vi "Untitled 1.vi"() -> ()   [LabVIEW 2018]
uses:
  <vilib>/Utility/file.llb/Read Delimited Spreadsheet (DBL).vi
  PublicSubVI/Class/Sig2MS/Sig2MS.lvclass
panel:
  in  "max":dbl
  in  "min":dbl
  in  "error in (no error)":errorcluster
  in  "File Path":path
  in  "tabCtrl":T1(tab)
  in  "scriptUpd":bool
  in  "Script":string
  out "rawGraph":cluster{"x":dbl[], "y":dbl[]}(graph)
  out "diffGraph":cluster{"x":dbl[], "y":dbl[]}(graph)
  out "diffSgolayGraph":cluster{"x":dbl[], "y":dbl[]}(graph)
  out "diffConvolveGraph":cluster{"x":dbl[], "y":dbl[]}(graph)
  out "richardsonGraph":cluster{"x":dbl[], "y":dbl[]}(graph)
  out "richardsonSgolayGraph":cluster{"x":dbl[], "y":dbl[]}(graph)
  out "richardsonConvolveGraph":cluster{"x":dbl[], "y":dbl[]}(graph)
  out "sgolayGraph":cluster{"x":dbl[], "y":dbl[]}(graph)
  out "sgolaySgolayGraph":cluster{"x":dbl[], "y":dbl[]}(graph)
  out "sgolayConvolveGraph":cluster{"x":dbl[], "y":dbl[]}(graph)
  out "sgolayAdvGraph":cluster{"x":dbl[], "y":dbl[]}(graph)
  out "sgolayAdvSgolayGraph":cluster{"x":dbl[], "y":dbl[]}(graph)
  out "sgolayAdvConvolveGraph":cluster{"x":dbl[], "y":dbl[]}(graph)
  out "xyGraph":cluster{"x":dbl[], "y":dbl[]}[](graph)
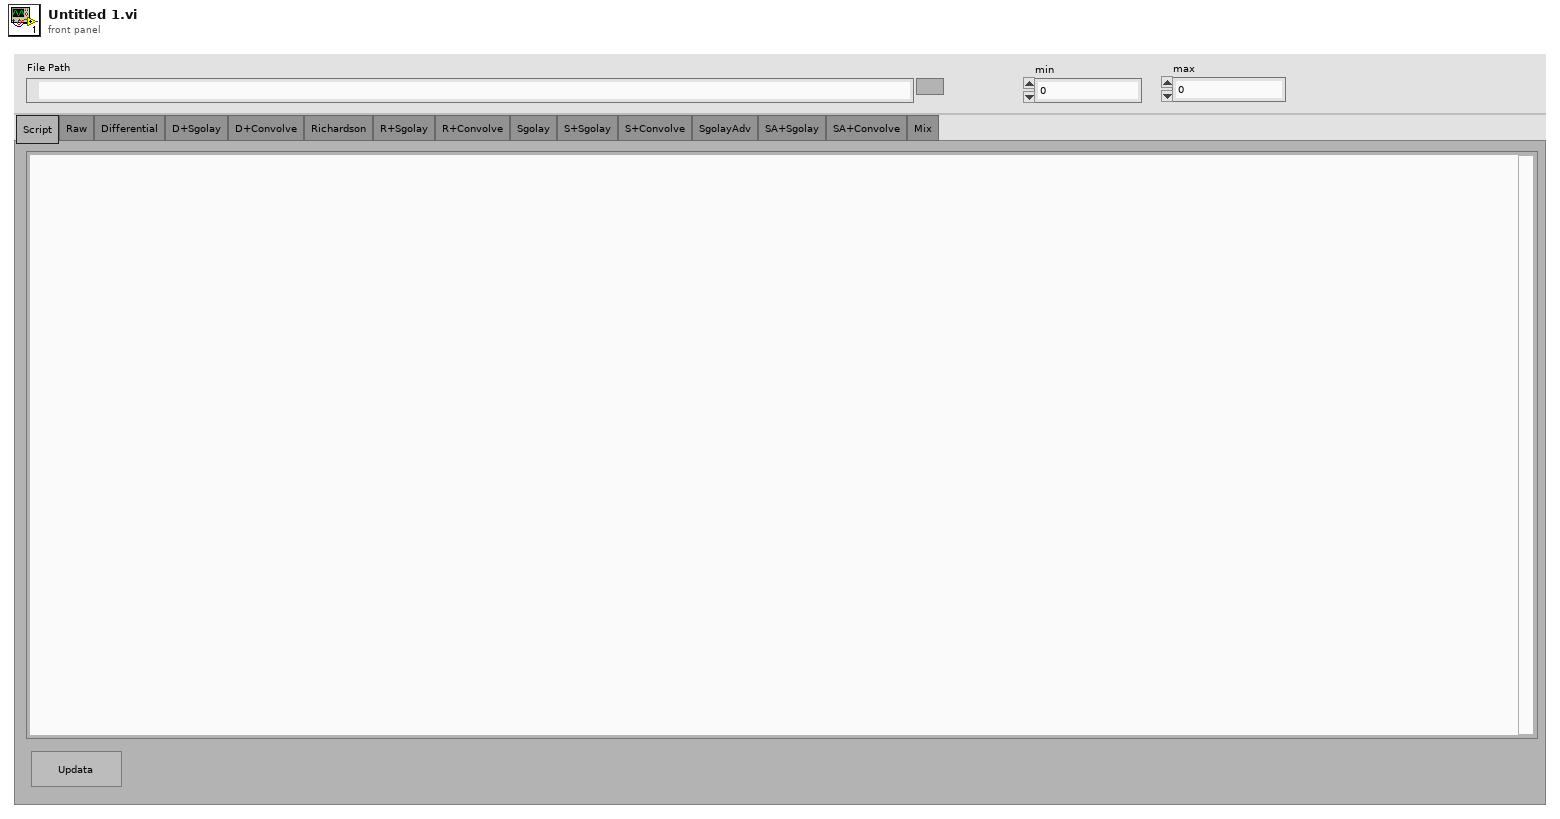
[diagram p1: front panel]
types:
  T1 = enum32{"Script", "Raw", "Differential", "D+Sgolay", "D+Convolve", "Richardson", "R+Sgolay", "R+Convolve", "Sgolay", "S+Sgolay", "S+Convolve", "SgolayAdv", "SA+Sgolay", "SA+Convolve", "Mix"}
  T2 = cluster{"startTime":dbl, "scanSig":cluster{"priDt":dbl, "priXData":dbl[], "priYData":sgl[], "beta":dbl[]}[], "ionSig":cluster{"secDt":dbl, "secYData":sgl[]}[]}
  T3 = enum16{"init", "loadScript", "newScript", "runScript", "close"}
  T4 = cluster{"priDt":dbl, "priXData":dbl[], "priYData":sgl[], "beta":dbl[]}[]
  T5 = cluster{"priDt":dbl, "priXData":dbl[], "priYData":sgl[], "beta":dbl[]}
  T6 = cluster{"startTime":dbl, "scanData":cluster{"dt":dbl, "xdata":dbl[], "ydata":sgl[], "beta":dbl[]}[], "xyXLabel":string, "xyYLabel":string, "wfmXLabel":string, "wfmYLabel":string, "ionData":cluster{"dt":dbl, "ydata":sgl[]}[], "ionXLabel":string, "ionYLabel":string}
  T7 = cluster{"dt":dbl, "xdata":dbl[], "ydata":sgl[], "beta":dbl[]}[]
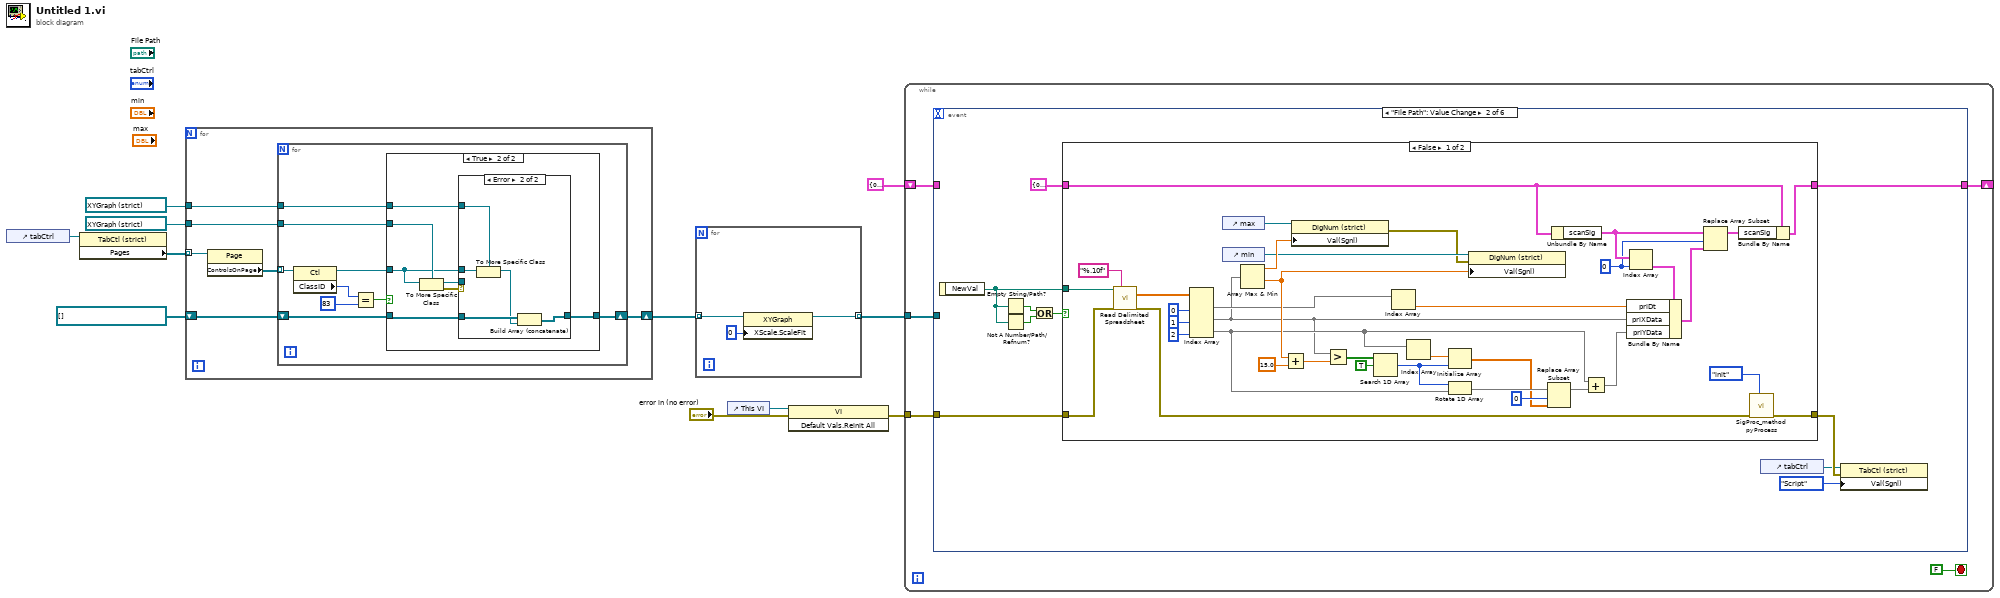
[diagram p0: block diagram]
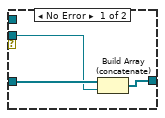
[diagram p3: hidden frame]
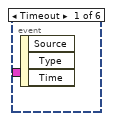
[diagram p4: hidden frame]
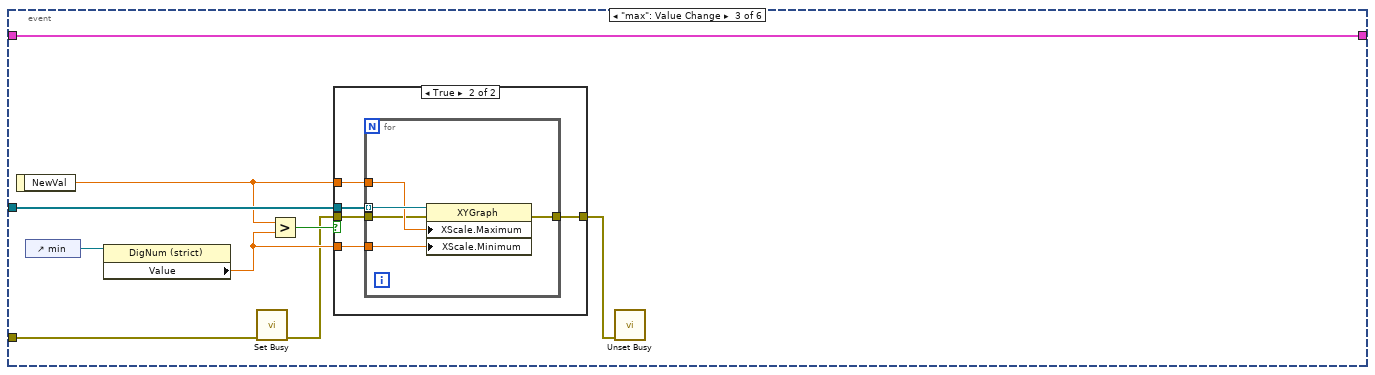
[diagram p6: hidden frame]
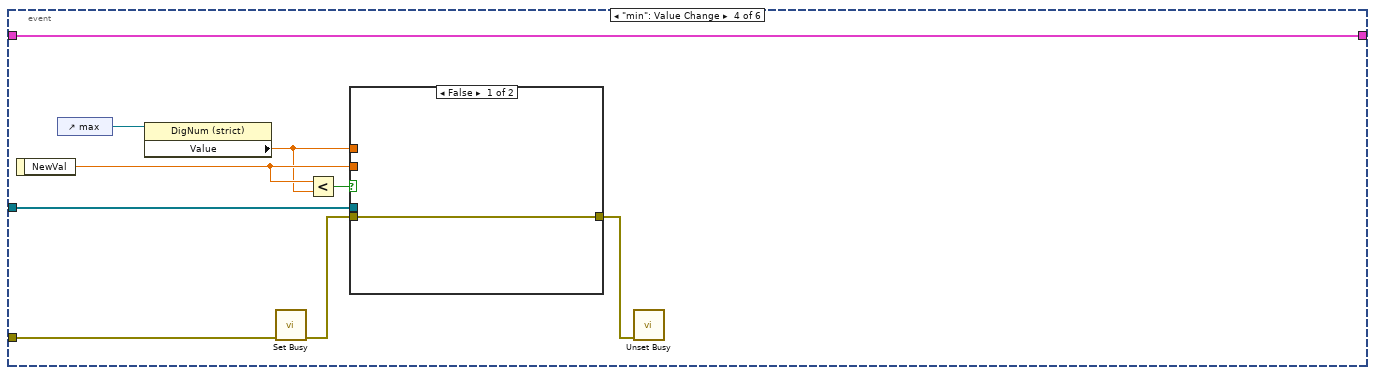
[diagram p8: hidden frame]
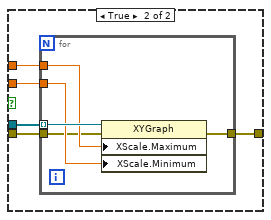
[diagram p9: hidden frame]
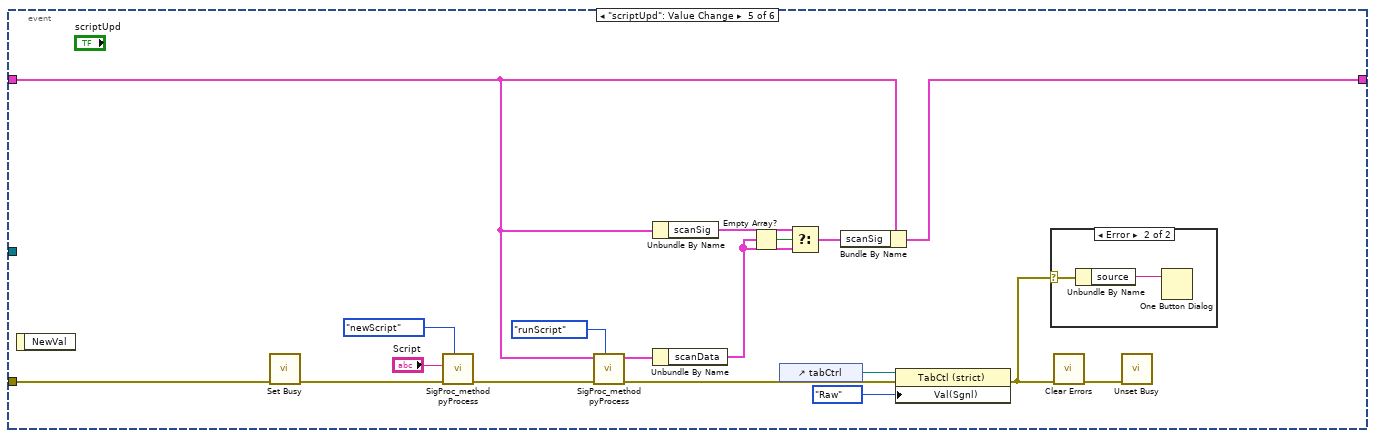
[diagram p10: hidden frame]
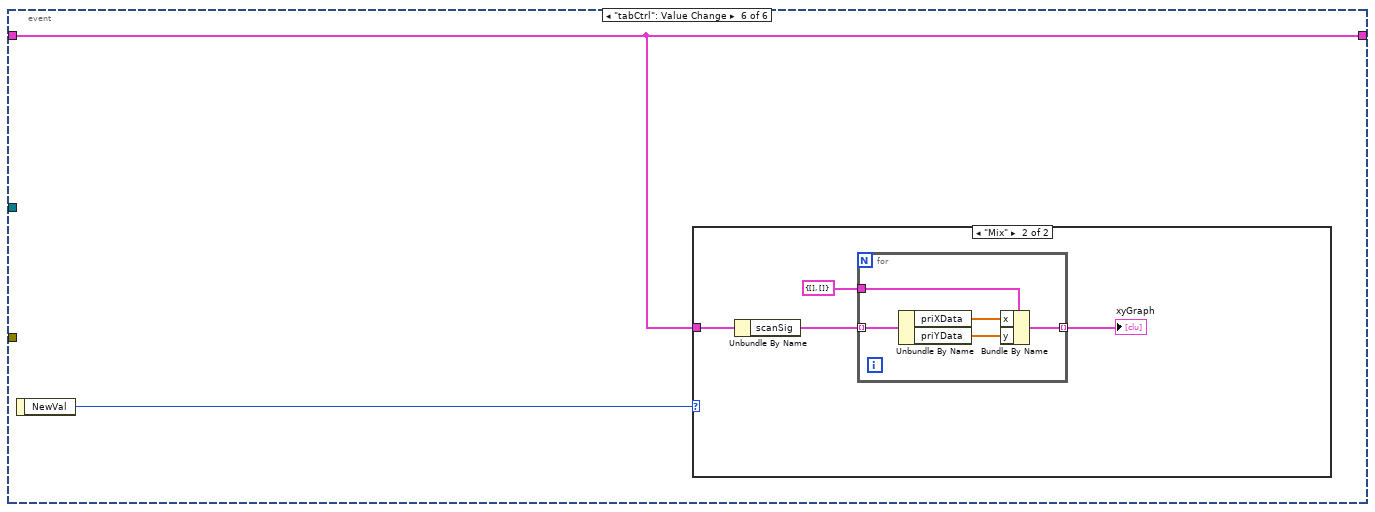
[diagram p12: hidden frame]
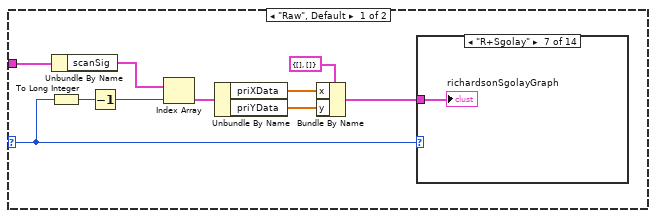
[diagram p13: hidden frame]
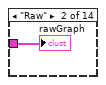
[diagram p15: hidden frame]
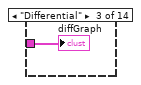
[diagram p16: hidden frame]
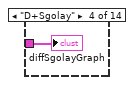
[diagram p17: hidden frame]
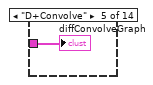
[diagram p18: hidden frame]
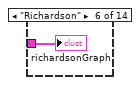
[diagram p19: hidden frame]
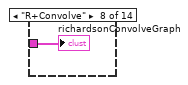
[diagram p20: hidden frame]
diagram:
  n1 = control-ref of="tabCtrl"() -> (w7:refnum<vi>)
  n2 = property class="TabCtl (strict)"(reference=w7) -> ("Pages"=w6:refnum<vi>[])  [unwired: 1 in, 2 out]
  n3 = for {
    tunnel: w6 -> [w17] mode=indexing
    shift-right: [w14] -> w2
    shift-left: refnum<vi>[] [] -> [w15]
    tunnel: refnum<vi> refnum ("diffGraph") -> [w13]
    tunnel: refnum<vi> refnum ("xyGraph") -> [w12]
    n4 = property class="Page"(reference=w17) -> ("ControlsOnPage"=w16:refnum<vi>[])  [unwired: 1 in, 2 out]
    n5 = for {
      tunnel: w16 -> [w26] mode=indexing
      shift-right: [w20] -> w14
      shift-left: w15 -> [w22]
      tunnel: w13 -> [w19]
      tunnel: w12 -> [w18]
      n6 = property class="Ctl"(reference=w26) -> (reference out=w21:refnum<vi>, "ClassID"=w25:u32)  [unwired: 1 in, 1 out]
      n7 = Equal?(x=w25, y=u32 83) -> (x = y?=w23:bool)
      n8 = case shown="True" w23 {
        tunnel: w22 -> [w27 w34]
        tunnel: w21 -> [_ w28]
        tunnel: [w27 w33] -> w20
        tunnel: w19 -> [_ w32]
        tunnel: w18 -> [_ w29]
        frame False {
        }
        frame True {
          n9 = To More Specific Class(target class=w32, reference=w28) -> (specific class reference=w31:refnum<vi>, error out=w30:errorcluster)  [unwired: 1 in]
          n10 = case shown="Error" w30 {
            tunnel: w34 -> [w37 w42]
            tunnel: [w36 w39] -> w33
            tunnel: w31 -> [w35 _]
            tunnel: w29 -> [_ w41]
            tunnel: w28 -> [_ w38]
            frame No Error {
              n11 = Build Array (concatenate)(w37, w35) -> (w36:refnum<vi>[])
            }
            frame Error {
              n12 = To More Specific Class(target class=w41, reference=w38) -> (specific class reference=w40:refnum<vi>)  [unwired: 1 in, 1 out]
              n13 = Build Array (concatenate)(w42, w40) -> (w39:refnum<vi>[])
            }
          }
        }
      }
    }
  }
  n14 = for {
    tunnel: w2 -> [w45] mode=indexing
    tunnel: [w44] -> w1 mode=indexing
    n15 = property class="XYGraph"(reference=w45, "XScale.ScaleFit"=u8 0 ("X Scale.Scale Fit")) -> (reference out=w44:refnum<vi>)  [unwired: 1 in, 1 out]
  }
  n16 = control-ref of="This VI"() -> (w8:refnum<vi>)
  n17 = invoke class="VI" method="Default Vals.Reinit All"(reference=w8, error in="error in (no error)") -> (error out=w10:errorcluster)  [unwired: 1 in, 2 out]
  n18 = while {
    shift-right: [w48] -> _
    shift-left: T2 {"startTime"=0.0, "scanSig"=[], "ionSig"=[]} ("dataParam") -> [w49]
    tunnel: w10 -> [w47]
    tunnel: w1 -> [w46]
    stop <- FALSE stop-if-true
    n19 = event shown="[1] \"File Path\": Value Change" {
      selector: _ -> [_ _ _ _ _ _]
      dyn-events: _ -> [_ _ _ _ _ _]
      timeout: _ -> [_ _ _ _ _ _]
      tunnel: w49 -> [_ _ w103 w123 w150 w161]
      tunnel: [_ w57 w103 w123 w152 w161] -> w48
      tunnel: w47 -> [_ w54 w102 w122 w145 _]
      tunnel: w46 -> [_ _ w107 w126 _ _]
      event Timeout {
        n20 = event-data() -> ()  [unwired: 1 in, 3 out]
      }
      event "File Path": Value Change {
        n21 = event-data() -> ("NewVal"=w56:path)  [unwired: 1 in]
        n22 = Empty String/Path?(string/path=w56) -> (empty?=w60:bool)
        n23 = Not A Number/Path/Refnum?(number/path/refnum=w56) -> (NaN/Path/Refnum?=w59:bool)
        n24 = Or(x=w60, y=w59) -> (x .or. y?=w58:bool)
        n25 = case shown="False" w58 {
          tunnel: T2 {"startTime"=0.0, "scanSig"=[{"priDt"=0.0, "priXData"=[], "priYData"=[], "beta"=[]}, {"priDt"=0.0, "priXData"=[], "priYData"=[], "beta"=[]}, {"priDt"=0.0, "priXData"=[], "priYData"=[], "beta"=[]}, {"priDt"=0.0, "priXData"=[], "priYData"=[], "beta"=[]}, {"priDt"=0.0, "priXData"=[], "priYData"=[], "beta"=[]}, {"priDt"=0.0, "priXData"=[], "priYData"=[], "beta"=[]}, {"priDt"=0.0, "priXData"=[], "priYData"=[], "beta"=[]}, {"priDt"=0.0, "priXData"=[], "priYData"=[], "beta"=[]}, {"priDt"=0.0, "priXData"=[], "priYData"=[], "beta"=[]}, {"priDt"=0.0, "priXData"=[], "priYData"=[], "beta"=[]}, {"priDt"=0.0, "priXData"=[], "priYData"=[], "beta"=[]}, {"priDt"=0.0, "priXData"=[], "priYData"=[], "beta"=[]}, {"priDt"=0.0, "priXData"=[], "priYData"=[], "beta"=[]}], "ionSig"=[]} ("dataParam") -> [w87 w99]
          tunnel: [w85 w99] -> w57
          tunnel: w56 -> [w93 _]
          tunnel: w54 -> [w91 w98]
          tunnel: [w66 w98] -> w53
          frame False {
            w89 = 0 ("index")
            n26 = call-poly <vilib>:"Read Delimited Spreadsheet.vi"("file path (dialog if empty)"=w93, "format (%.3f)"="%.10f", "error in (no error)"=w91) -> ("all rows"=w97:dbl[][], "error out"=w67:errorcluster)  [unwired: 7 in, 4 out]
            n27 = Index Array(array=w97, index (col) #1=0 ("disabled index (col)"), index (col) #2=1 ("index (col)"), index (col) #3=2 ("index (col)")) -> (element #1=w62:dbl[], element #2=w61:dbl[], element #3=w64:dbl[])  [unwired: 3 in]
            n28 = control-ref of="max"() -> (w83:refnum<vi>)
            n29 = control-ref of="min"() -> (w82:refnum<vi>)
            n30 = Array Max & Min(array=w61) -> (max value=w84:dbl, min value=w74:dbl)  [unwired: 2 out]
            n31 = Add(x=w74, y=15.0) -> (x+y=w69:dbl)
            n32 = property class="DigNum (strict)"(reference=w83, "Val(Sgnl)"=w84) -> (error out=w81:errorcluster)  [unwired: 1 in, 1 out]
            n33 = Greater?(x=w61, y=w69) -> (0:w72:bool[])
            n34 = Search 1D Array(1D array=w72, element=TRUE) -> (index of element=w70:i32)  [unwired: 1 in]
            n35 = Index Array(array=w62) -> (element=w63:dbl)  [unwired: 1 in]
            n36 = Index Array(array=w64) -> (element=w75:dbl)  [unwired: 1 in]
            n37 = Initialize Array(w75, w70) -> (w78:dbl[])
            n38 = Rotate 1D Array(1:w64, 2:w70) -> (0:w80:dbl[])
            n39 = property class="DigNum (strict)"(reference=w82, error in=w81, "Val(Sgnl)"=w74) -> ()  [unwired: 2 out]
            n40 = Replace Array Subset(array=w80, new element=w78, index=0) -> (w77:dbl[])
            n41 = Unbundle By Name(w87) -> ("scanSig"=w90:T4)
            n42 = Add(x=w64, y=w77) -> (x+y=w76:dbl[])
            n43 = Index Array(array=w90, index=w89) -> (element=w92:T5)
            n44 = Bundle By Name(cluster=w92, "priDt"=w63, "priXData"=w61, "priYData"=w76) -> (w88:T5)
            n45 = Replace Array Subset(array=w90, new element=w88, index=w89) -> (w86:T4)
            n46 = Bundle By Name(cluster=w87, "scanSig"=w86) -> (w85:T2)
            n47 = call "SigProc_method pyProcess.vi"("func"=T3."init", "error in (no error)"=w67) -> ("error out"=w66:errorcluster)  [unwired: 6 in, 3 out]
          }
          frame True {
          }
        }
        n48 = control-ref of="tabCtrl"() -> (w51:refnum<vi>)
        n49 = property class="TabCtl (strict)"(reference=w51, error in=w53, "Val(Sgnl)"=T1."Script" ("Value (Signaling)")) -> ()  [unwired: 2 out]
      }
      event "max": Value Change {
        n50 = event-data() -> ("NewVal"=w104:dbl)  [unwired: 1 in]
        n51 = control-ref of="min"() -> (w106:refnum<vi>)
        n52 = property class="DigNum (strict)"(reference=w106) -> ("Value"=w105:dbl)  [unwired: 1 in, 2 out]
        n53 = call <vilib>:"Set Busy.vi"("error in (no error)"=w102) -> ("error out"=w101:errorcluster)  [unwired: 9 in, 1 out]
        n54 = Greater?(x=w104, y=w105) -> (0:w108:bool)
        n55 = case shown="True" w108 {
          tunnel: w107 -> [_ w114]
          tunnel: w104 -> [_ w113]
          tunnel: w105 -> [_ w112]
          tunnel: w101 -> [w109 w111]
          tunnel: [w109 w110] -> w100
          frame False {
          }
          frame True {
            n56 = for {
              tunnel: w114 -> [w119] mode=indexing
              tunnel: w113 -> [w118]
              tunnel: w112 -> [w117]
              tunnel: w111 -> [w116]
              tunnel: [w115] -> w110
              n57 = property class="XYGraph"(reference=w119, error in=w116, "XScale.Maximum"=w118, "XScale.Minimum"=w117) -> (error out=w115:errorcluster)  [unwired: 1 out]
            }
          }
        }
        n58 = call <vilib>:"Unset Busy.vi"("error in (no error)"=w100) -> ()  [unwired: 10 in, 1 out]
      }
      event "min": Value Change {
        n59 = event-data() -> ("NewVal"=w125:dbl)  [unwired: 1 in]
        n60 = control-ref of="max"() -> (w128:refnum<vi>)
        n61 = property class="DigNum (strict)"(reference=w128) -> ("Value"=w124:dbl)  [unwired: 1 in, 2 out]
        n62 = call <vilib>:"Set Busy.vi"("error in (no error)"=w122) -> ("error out"=w121:errorcluster)  [unwired: 9 in, 1 out]
        n63 = Less?(x=w125, y=w124) -> (x < y?=w127:bool)
        n64 = case shown="False" w127 {
          tunnel: w126 -> [_ w134]
          tunnel: w125 -> [_ w132]
          tunnel: w124 -> [_ w133]
          tunnel: w121 -> [w129 w131]
          tunnel: [w129 w130] -> w120
          frame False {
          }
          frame True {
            n65 = for {
              tunnel: w134 -> [w139] mode=indexing
              tunnel: w133 -> [w138]
              tunnel: w132 -> [w137]
              tunnel: w131 -> [w136]
              tunnel: [w135] -> w130
              n66 = property class="XYGraph"(reference=w139, error in=w136, "XScale.Maximum"=w138, "XScale.Minimum"=w137) -> (error out=w135:errorcluster)  [unwired: 1 out]
            }
          }
        }
        n67 = call <vilib>:"Unset Busy.vi"("error in (no error)"=w120) -> ()  [unwired: 10 in, 1 out]
      }
      event "scriptUpd": Value Change {
        n68 = event-data() -> ()  [unwired: 1 in, 1 out]
        n69 = call <vilib>:"Set Busy.vi"("error in (no error)"=w145) -> ("error out"=w144:errorcluster)  [unwired: 9 in, 1 out]
        n70 = call "SigProc_method pyProcess.vi"("func"=T3."newScript", "error in (no error)"=w144, "newScriptCode"="Script") -> ("error out"=w157:errorcluster)  [unwired: 5 in, 3 out]
        n71 = call "SigProc_method pyProcess.vi"("func"=T3."runScript", "error in (no error)"=w157, "dataParam"=w150) -> ("error out"=w151:errorcluster, "newSigInfo"=w153:T6)  [unwired: 5 in, 2 out]
        n72 = Unbundle By Name(w150) -> ("scanSig"=w149:T4)
        n73 = Unbundle By Name(w153) -> ("scanData"=w147:T7)
        n74 = Empty Array?(array=w147) -> (empty?=w146:bool)
        n75 = control-ref of="tabCtrl"() -> (w141:refnum<vi>)
        n76 = Select(t=w149, s=w146, f=w147) -> (s? t:f=w148:T7)
        n77 = Bundle By Name(cluster=w150, "scanSig"=w148) -> (w152:T2)
        n78 = property class="TabCtl (strict)"(reference=w141, error in=w151, "Val(Sgnl)"=T1."Raw" ("Value (Signaling)")) -> (error out=w140:errorcluster)  [unwired: 1 out]
        n79 = case shown="Error" w140 {
          selector: w140 -> [_ w158]
          frame No Error {
          }
          frame Error {
            n80 = Unbundle By Name(w158) -> ("source"=w159:string)
            n81 = One Button Dialog(message=w159) -> ()  [unwired: 1 in, 1 out]
          }
        }
        n82 = call <vilib>:"Clear Errors.vi"("error in (no error)"=w140) -> ("error out"=w143:errorcluster)  [unwired: 5 in, 1 out]
        n83 = call <vilib>:"Unset Busy.vi"("error in (no error)"=w143) -> ()  [unwired: 10 in, 1 out]
      }
      event "tabCtrl": Value Change {
        n84 = event-data() -> ("NewVal"=w160:T1)  [unwired: 1 in]
        n85 = case shown="\"Mix\"" w160 {
          selector: w160 -> [w163 _]
          tunnel: w161 -> [w164 w188]
          frame "Raw", Default {
            n86 = To Long Integer(number=w163) -> (32bit integer=w166:i32)
            n87 = Unbundle By Name(w164) -> ("scanSig"=w171:T4)
            n88 = Decrement(x=w166) -> (x-1=w165:i32)
            n89 = Index Array(array=w171, index=w165) -> (element=w170:T5)
            n90 = Unbundle By Name(w170) -> ("priXData"=w168:dbl[], "priYData"=w167:sgl[])
            n91 = Bundle By Name(cluster=cluster{"x":dbl[], "y":dbl[]} {"x"=[], "y"=[]} ("Value"), "x"=w168, "y"=w167) -> (w162:cluster{"x":dbl[], "y":dbl[]})
            n92 = case shown="\"R+Sgolay\"" w163 {
              tunnel: w162 -> [_ w172 w173 w174 w175 w176 w177 w178 w179 w180 w181 w182 w183 w184]
              frame "Script", Default {
              }
              frame "Raw" {
                "rawGraph" <- w172
              }
              frame "Differential" {
                "diffGraph" <- w173
              }
              frame "D+Sgolay" {
                "diffSgolayGraph" <- w174
              }
              frame "D+Convolve" {
                "diffConvolveGraph" <- w175
              }
              frame "Richardson" {
                "richardsonGraph" <- w176
              }
              frame "R+Sgolay" {
                "richardsonSgolayGraph" <- w177
              }
              frame "R+Convolve" {
                "richardsonConvolveGraph" <- w178
              }
              frame "Sgolay" {
                "sgolayGraph" <- w179
              }
              frame "S+Sgolay" {
                "sgolaySgolayGraph" <- w180
              }
              frame "S+Convolve" {
                "sgolayConvolveGraph" <- w181
              }
              frame "SgolayAdv" {
                "sgolayAdvGraph" <- w182
              }
              frame "SA+Sgolay" {
                "sgolayAdvSgolayGraph" <- w183
              }
              frame "SA+Convolve" {
                "sgolayAdvConvolveGraph" <- w184
              }
            }
          }
          frame "Mix" {
            n93 = Unbundle By Name(w188) -> ("scanSig"=w187:T4)
            n94 = for {
              tunnel: w187 -> [w189] mode=indexing
              tunnel: [w191] -> w186 mode=indexing
              tunnel: cluster{"x":dbl[], "y":dbl[]} {"x"=[], "y"=[]} ("Value") -> [w190]
              n95 = Unbundle By Name(w189) -> ("priXData"=w193:dbl[], "priYData"=w192:sgl[])
              n96 = Bundle By Name(cluster=w190, "x"=w193, "y"=w192) -> (w191:cluster{"x":dbl[], "y":dbl[]})
            }
            "xyGraph" <- w186
          }
        }
      }
    }
  }
